vi "pRUEBA2_VERSION2_2.vi"() -> ()   [LabVIEW 2013]
panel:
  out "Mucha calor":bool
  out "Temperatura Mayor":dbl
  out "Contador":dbl
  out "TempPromedio":dbl
  out "Thermometer":i32(slide) scale=0.0..60.0
  # "SE TIENE QUE GENERAR LA TEMPERATURA DE TODO UN DÍA EN INTERVALOS DE DOS HORAS\nAL FINAL DEL DÍA DEBERÁN DE PRESENTAR LA TEMPERATURA PROMEDIO DE LAS\nTEMPERATURAS MAYORES A 35 GRADOS Y CONTARLAS\nAL FINAL DE DÍA PRESENTAR LA TEMPERATURA MAYOR\nCUANDO LA TEMPERATURA EXCEDA LOS 40 GRADOS DEBERÁ DE ENCENDER UN LED.\nEL PROGRAMA PUEDE DETENERSE SI HAY UNA TEMPERATURA ARRIBA DE LOS 55\nGRADOS"
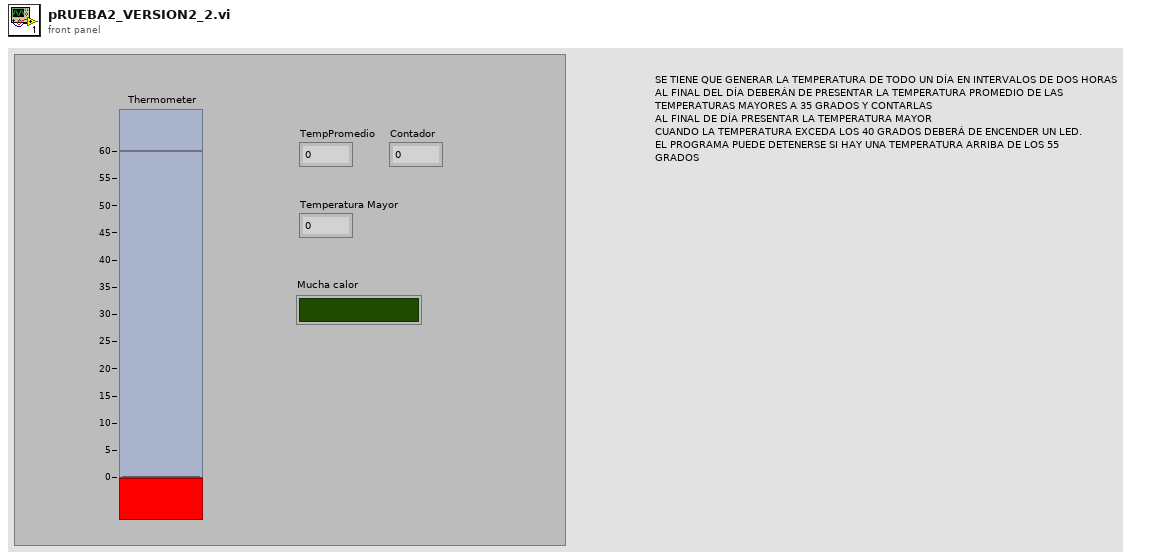
[diagram p1: front panel]
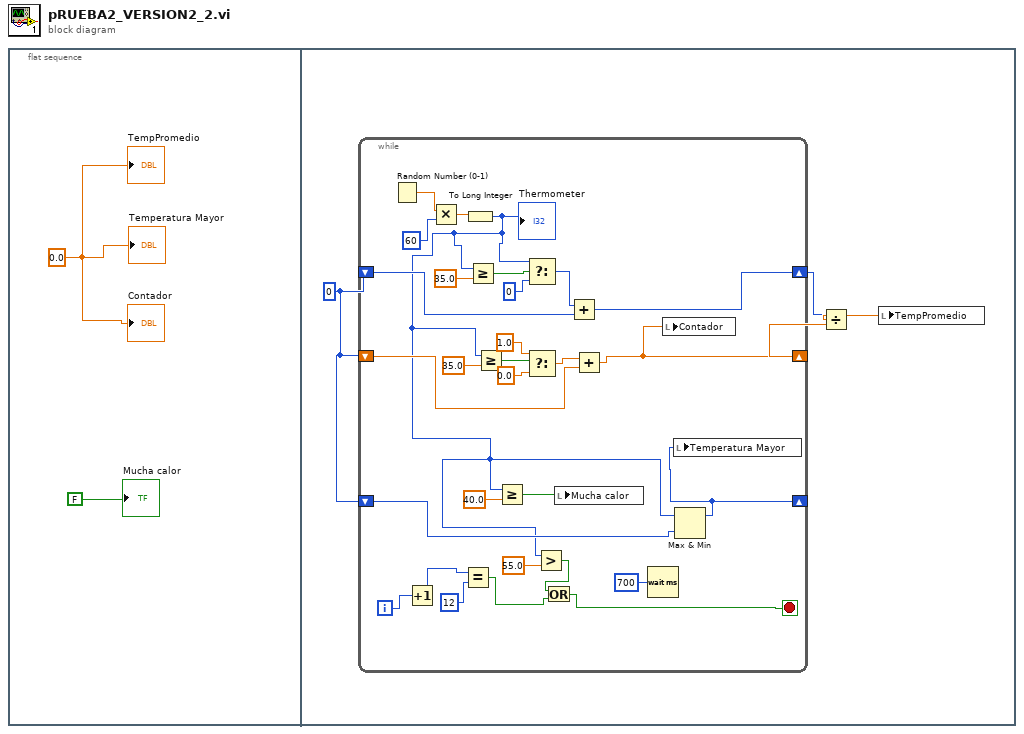
[diagram p0: block diagram]
diagram:
  n1 = flat-sequence {
    frame #0 {
      w2 = 0.0 ("Temperatura Mayor")
      "TempPromedio" <- w2
      "Temperatura Mayor" <- w2
      "Contador" <- w2
      "Mucha calor" <- FALSE
    }
    frame #1 {
      w4 = 0
      n2 = while {
        shift-right: [w27] -> w3
        shift-left: w4 -> [w29]
        shift-right: [w20] -> w6
        shift-left: w4 -> [w21]
        shift-right: [w16] -> _
        shift-left: w4 -> [w17]
        i -> [w14]
        stop <- w7 stop-if-true
        n3 = Random Number (0-1)() -> (number: 0 to 1=w34:dbl)
        n4 = Increment(x=w14) -> (x+1=w13:i32)
        n5 = Multiply(x=w34, y=60) -> (x*y=w33:dbl)
        n6 = Equal?(x=w13, y=12) -> (x = y?=w8:bool)
        n7 = To Long Integer(number=w33) -> (32bit integer=w10:i32)
        "Thermometer" <- w10
        n8 = Greater Or Equal?(x=w10, y=35.0) -> (x >= y?=w31:bool)
        n9 = Greater Or Equal?(x=w10, y=35.0) -> (x >= y?=w26:bool)
        n10 = Greater Or Equal?(x=w10, y=40.0) -> (x >= y?=w18:bool)
        n11 = Select(t=w10, s=w31, f=0) -> (s? t:f=w28:i32)
        n12 = Select(t=1.0, s=w26, f=0.0) -> (s? t:f=w22:dbl)
        n13 = Greater?(x=w10, y=55.0) -> (0:w9:bool)
        n14 = Or(x=w9, y=w8) -> (x .or. y?=w7:bool)
        n15 = local write "Mucha calor"(w18) -> ()
        n16 = Add(x=w28, y=w29) -> (x+y=w27:i32)
        n17 = Add(x=w22, y=w21) -> (x+y=w20:dbl)
        n18 = Wait (ms)(milliseconds to wait=u32 700) -> ()  [unwired: 1 out]
        n19 = local write "Contador"(w20) -> ()
        n20 = Max & Min(x=w10, y=w17) -> (max(x,y)=w16:i32)  [unwired: 1 out]
        n21 = local write "Temperatura Mayor"(w16) -> ()
      }
      n22 = Divide(x=w3, y=w6) -> (x/y=w5:dbl)
      n23 = local write "TempPromedio"(w5) -> ()
    }
  }
